vi "SodaDispenserRobot.vi"() -> ()   [LabVIEW 2018]
uses:
  <vilib>/Instr/_visa.llb/VISA Configure Serial Port (Instr).vi
panel:
  in  "?":bool
  in  "?":bool
  in  "?":bool
  # "COCA COLA"
  # "SPRITE"
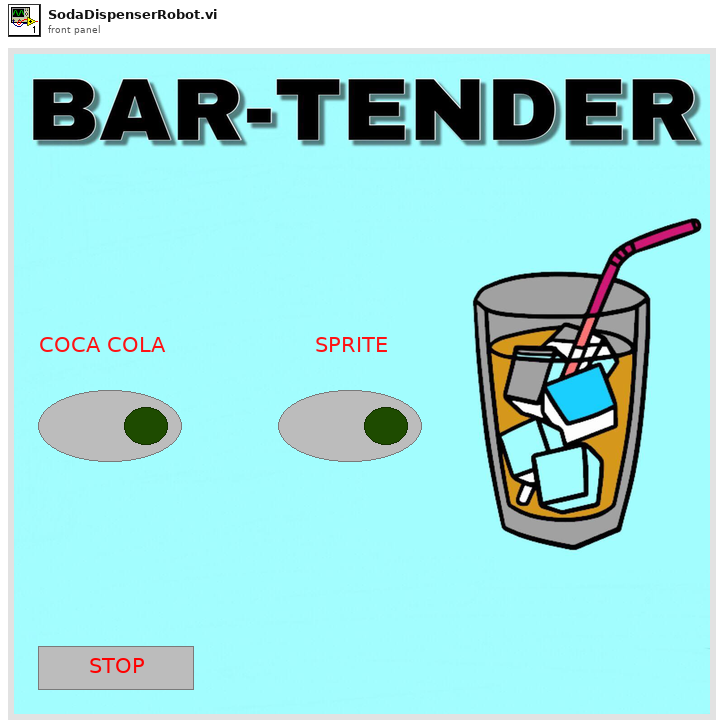
[diagram p1: front panel]
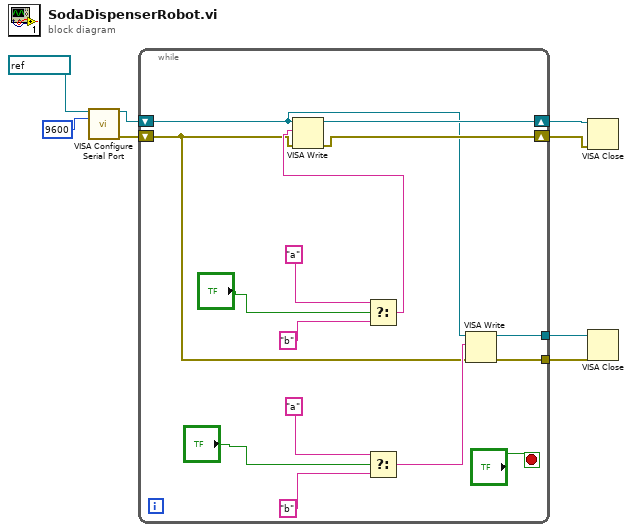
[diagram p0: block diagram]
diagram:
  n1 = call-poly "VISA Configure Serial Port"("VISA resource name"=refnum<visa-resource-name> "COM4", "baud rate (9600)"=u32 9600) -> ("VISA resource name out"=w7:refnum<visa-resource-name>, "error out"=w6:errorcluster)  [unwired: 12 in]
  n2 = while {
    tunnel: [w13] -> w3
    tunnel: [w12] -> w2
    shift-right: [w20] -> w4
    shift-left: w7 -> [w15]
    shift-right: [w21] -> w5
    shift-left: w6 -> [w14]
    stop <- "?" stop-if-true
    n3 = Select(t="a", s="?", f="b") -> (s? t:f=w19:string)
    n4 = VISA Write(VISA resource name=w15, write buffer=w19, error in (no error)=w14) -> (VISA resource name out=w20:refnum<visa-resource-name>, error out=w21:errorcluster)  [unwired: 1 out]
    n5 = Select(t="a", s="?", f="b") -> (s? t:f=w16:string)
    n6 = VISA Write(VISA resource name=w15, write buffer=w16, error in (no error)=w14) -> (VISA resource name out=w13:refnum<visa-resource-name>, error out=w12:errorcluster)  [unwired: 1 out]
  }
  n7 = VISA Close(VISA resource name=w4, error in (no error)=w5) -> ()  [unwired: 1 out]
  n8 = VISA Close(VISA resource name=w3, error in (no error)=w2) -> ()  [unwired: 1 out]
